vi "normal_Flow.vi"(8 "error in":errorcluster, 11 "VISA resource name":refnum<visa-resource-name>="ASRL2::INSTR") -> (0 "error out":errorcluster, 3 "VISA resource out":refnum<visa-resource-name>="ASRL2::INSTR")   [LabVIEW 2010]
panel:
  in  "Action 2":u8(ring) items=["TurnON_1"=8, "TurnON_PUMP"=9, "TurnON_3"=10, "TurnON_4"=11, "CLOSE DUMP OFF_1"=0, "TurnOFF_PUMP"=1, "TurnOFF_3"=2, "TurnOFF_4"=3, "OpenAll"=30, "CloseAllRelay"=29]
  in  "Action":u8(ring) items=["TurnON_1"=8, "TurnON_PUMP"=9, "TurnON_3"=10, "TurnON_4"=11, "CLOSE DUMP OFF_1"=0, "TurnOFF_PUMP"=1, "TurnOFF_3"=2, "TurnOFF_4"=3, "OpenAll"=30, "CloseAllRelay"=29]
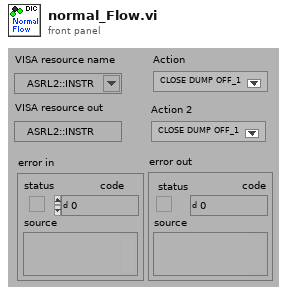
[diagram p1: front panel]
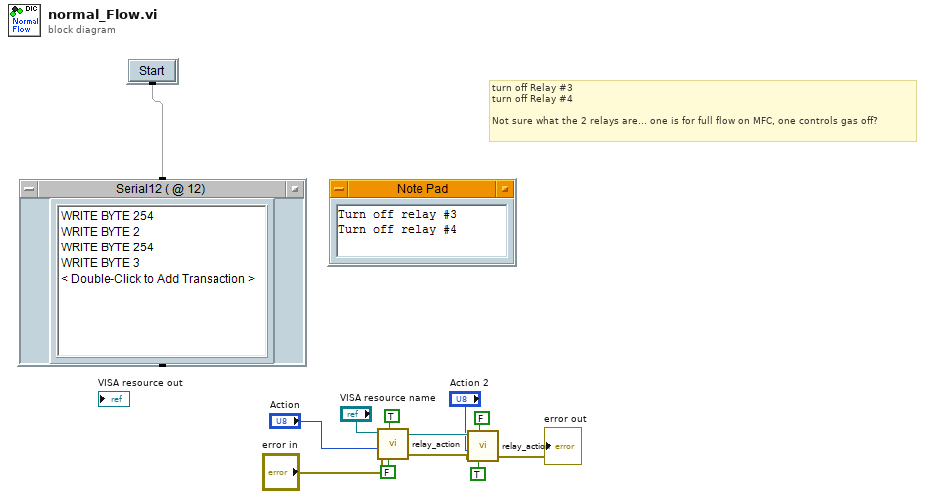
[diagram p0: block diagram]
diagram:
  # "turn off Relay #3\nturn off Relay #4\n\nNot sure what the 2 relays are... one is for full flow on MFC, one controls gas off?"
  n1 = call "relay_action.vi"("VISA resource name"="VISA resource name", "init?"=TRUE, "Action"="Action", "Quit?"=FALSE, "error in"="error in") -> ("VISA resource name 2"=w4:refnum<visa-resource-name>, "error out"=w3:errorcluster)  [unwired: 2 in]
  n2 = call "relay_action.vi"("VISA resource name"=w4, "init?"=FALSE, "Action"="Action 2", "Quit?"=TRUE, "error in"=w3) -> ("error out"=→"error out":errorcluster)  [unwired: 2 in, 1 out]
